vi "validate-warning.vi"(8 "max1":i16, 9 "min1":i16, 10 "war":i32, 11 "val":u16) -> (3 "status":bool)   [LabVIEW 2014]
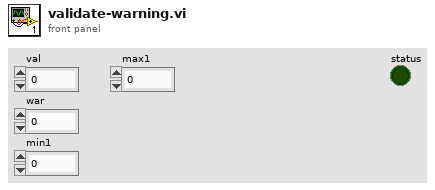
[diagram p1: front panel]
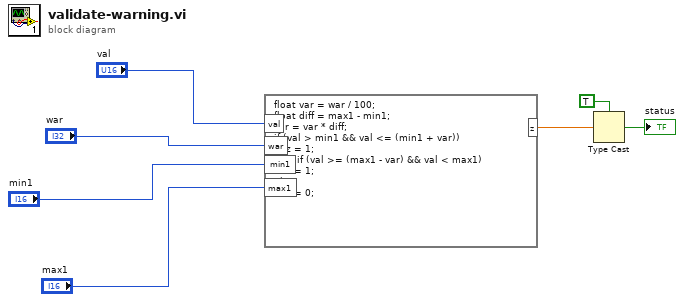
[diagram p0: block diagram]
diagram:
  n1 = formula code="float var = war / 100;\nfloat diff = max1 - min1;\nvar = var * diff;\nif (val > min1 && val <= (min1 + var))\n    z = 1;\nelse if (val >= (max1 - var) && val < max1)\n    z = 1;\nelse\n    z = 0;"("val"="val", "war"="war", "min1"="min1", "max1"="max1") -> ("z"=w2:dbl)
  n2 = Type Cast(type=TRUE, x=w2) -> (*(type *) &x=→"status":bool)
